vi "Get Fit Parameter Names, Values & Uncertainties.vi"(8 "error in (no error)":errorcluster, 9 "Fit Parameter Uncertainties":variant, 11 "Fit Parameters":variant) -> (0 "Error Out":errorcluster, 1 "Fit Parameter Uncertainties":dbl[](array[numeric]), 2 "Fit Parameter Values":dbl[](array[numeric]), 3 "Fit Parameter Names":string[](array[string]))   [LabVIEW 2019]
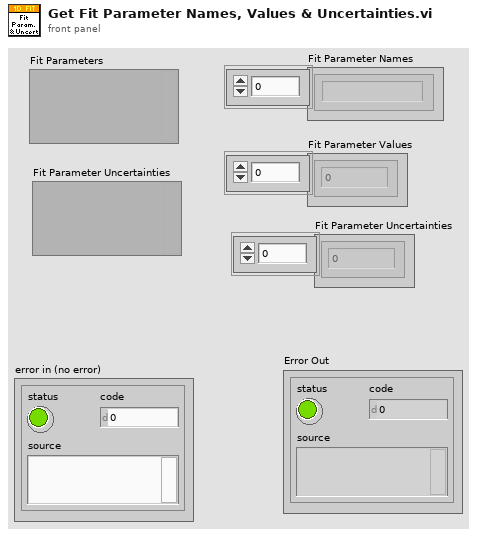
[diagram p1: front panel]
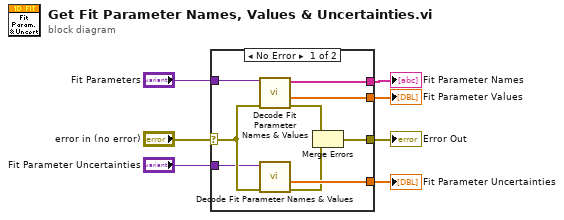
[diagram p0: block diagram]
diagram:
  n1 = case shown="No Error" "error in (no error)" {
    selector: "error in (no error)" -> [w12 w17]
    tunnel: [w16 _] -> w7
    tunnel: [w15 _] -> w6
    tunnel: "Fit Parameters" -> [w14 _]
    tunnel: [w13 w17] -> w4
    tunnel: [w11 _] -> w2
    tunnel: "Fit Parameter Uncertainties" -> [w10 _]
    frame No Error {
      n2 = call "Decode Fit Parameter Names & Values.vi"("Error In"=w12, "Fit Parameters"=w14) -> ("Error Out"=w9:errorcluster, "Parameter Values"=w16:dbl[], "Parameter Names"=w15:string[])  [unwired: 7 in]
      n3 = call "Decode Fit Parameter Names & Values.vi"("Error In"=w12, "Fit Parameters"=w10) -> ("Error Out"=w8:errorcluster, "Parameter Values"=w11:dbl[])  [unwired: 7 in, 1 out]
      n4 = Merge Errors(w9, w8) -> (w13:errorcluster)
    }
    frame Error {
    }
  }
  "Fit Parameter Values" <- w7
  "Fit Parameter Names" <- w6
  "Error Out" <- w4
  "Fit Parameter Uncertainties" <- w2
